vi "Trama_GGA(SubVI).vi"(0 "TRAMA":string) -> (1 "Cluster 2":T2, 2 "Cluster":T3, 3 "output":T1)   [LabVIEW 2020]
panel:
  out "String":string
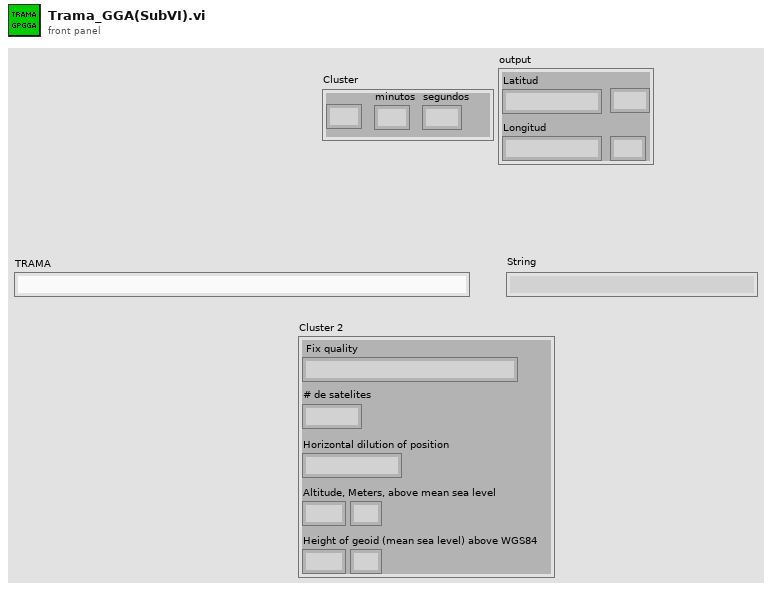
[diagram p1: front panel]
types:
  T1 = cluster{"Latitud":string, string, "Longitud":string, string}
  T2 = cluster{" Fix quality":string, "Horizontal dilution of position":string, "Altitude, Meters, above mean sea level":string, string, "Height of geoid (mean sea level) above WGS84":string, string, "# de satelites":string}
  T3 = cluster{"horas":string, "minutos":string, "segundos ":string}
  T4 = cluster{string, string, string, string, string, string, string}
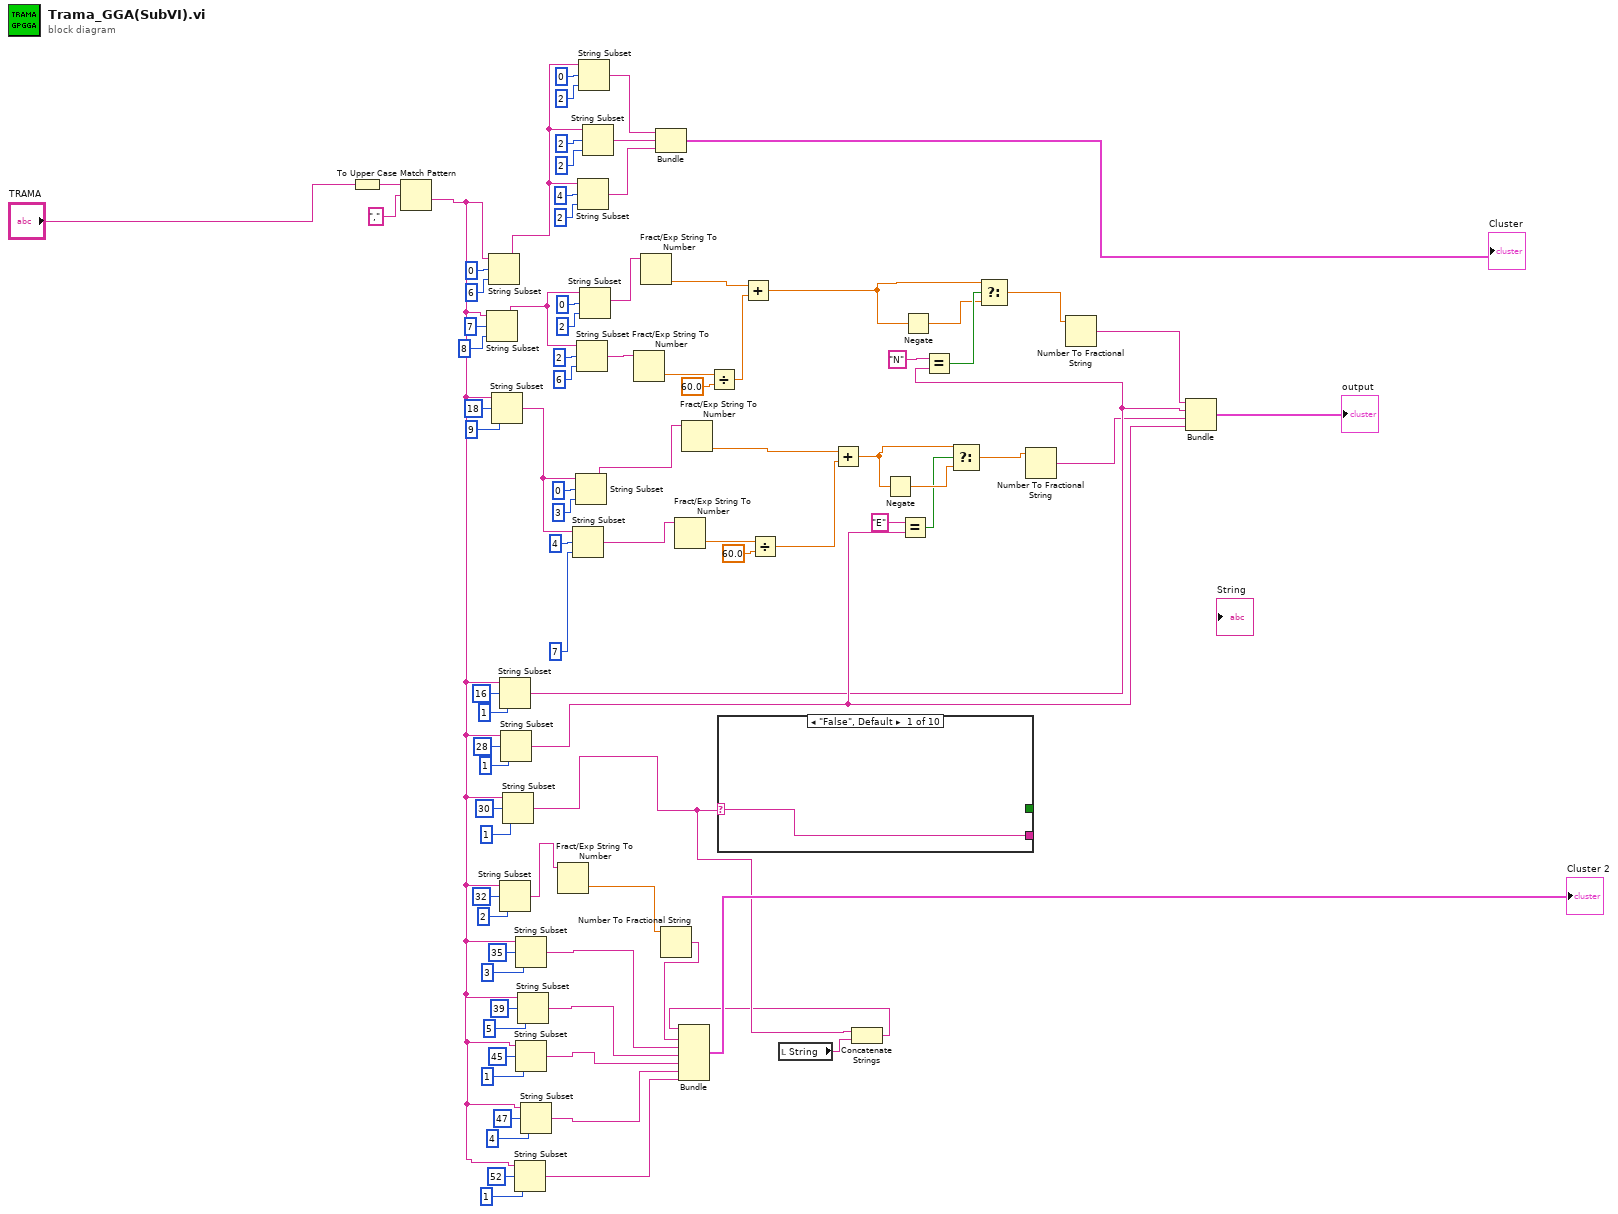
[diagram p0: block diagram]
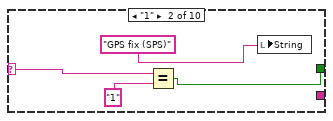
[diagram p2: hidden frame]
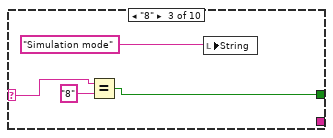
[diagram p3: hidden frame]
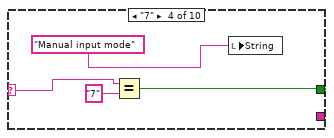
[diagram p4: hidden frame]
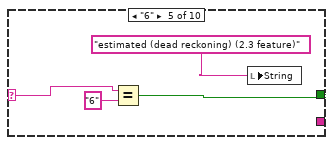
[diagram p5: hidden frame]
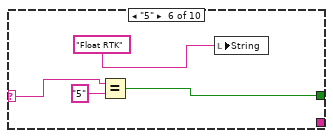
[diagram p6: hidden frame]
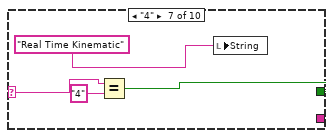
[diagram p7: hidden frame]
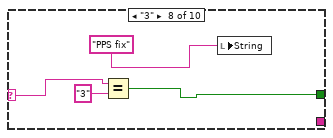
[diagram p8: hidden frame]
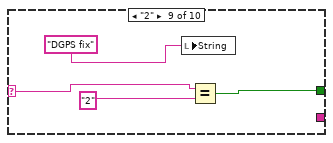
[diagram p9: hidden frame]
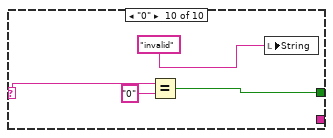
[diagram p10: hidden frame]
diagram:
  n1 = To Upper Case(1:"TRAMA") -> (0:w38:string)
  n2 = Match Pattern(string=w38, regular expression=",") -> (after substring=w80:string)  [unwired: 1 in, 3 out]
  n3 = String Subset(string=w80, offset (0)=7, length (rest)=8 ("length (rest)")) -> (substring=w35:string)
  n4 = String Subset(string=w80, offset (0)=0, length (rest)=6 ("length (rest)")) -> (substring=w37:string)
  n5 = String Subset(string=w80, offset (0)=18, length (rest)=9 ("length (rest)")) -> (substring=w51:string)
  n6 = String Subset(string=w80, offset (0)=16, length (rest)=1 ("length (rest)")) -> (substring=w58:string)
  n7 = String Subset(string=w80, offset (0)=32, length (rest)=2 ("length (rest)")) -> (substring=w87:string)
  n8 = String Subset(string=w80, offset (0)=28, length (rest)=1 ("length (rest)")) -> (substring=w65:string)
  n9 = String Subset(string=w80, offset (0)=30, length (rest)=1 ("length (rest)")) -> (substring=w10:string)
  n10 = String Subset(string=w80, offset (0)=52, length (rest)=1 ("length (rest)")) -> (substring=w85:string)
  n11 = String Subset(string=w80, offset (0)=35, length (rest)=3 ("length (rest)")) -> (substring=w81:string)
  n12 = String Subset(string=w80, offset (0)=45, length (rest)=1 ("length (rest)")) -> (substring=w83:string)
  n13 = String Subset(string=w80, offset (0)=39, length (rest)=5 ("length (rest)")) -> (substring=w82:string)
  n14 = String Subset(string=w80, offset (0)=47, length (rest)=4 ("length (rest)")) -> (substring=w84:string)
  n15 = Fract/Exp String To Number(string=w87) -> (number=w2:dbl)  [unwired: 3 in, 1 out]
  n16 = String Subset(string=w51, offset (0)=4, length (rest)=7 ("length (rest)")) -> (substring=w43:string)
  n17 = String Subset(string=w51, offset (0)=0, length (rest)=3 ("length (rest)")) -> (substring=w48:string)
  n18 = String Subset(string=w35, offset (0)=2, length (rest)=6 ("length (rest)")) -> (substring=w22:string)
  n19 = String Subset(string=w37, offset (0)=4, length (rest)=2 ("length (rest)")) -> (substring=w34:string)
  n20 = String Subset(string=w37, offset (0)=0, length (rest)=2 ("length (rest)")) -> (substring=w32:string)
  n21 = String Subset(string=w35, offset (0)=0, length (rest)=2 ("length (rest)")) -> (substring=w25:string)
  n22 = String Subset(string=w37, offset (0)=2, length (rest)=2 ("length (rest)")) -> (substring=w33:string)
  n23 = Fract/Exp String To Number(string=w22) -> (number=w23:dbl)  [unwired: 3 in, 1 out]
  n24 = Fract/Exp String To Number(string=w25) -> (number=w27:dbl)  [unwired: 3 in, 1 out]
  n25 = Bundle(w32, w33, w34) -> (→"Cluster":cluster{string, string, string})  [unwired: 1 in]
  n26 = Number To Fractional String(number=w2) -> (F-format string=w1:string)  [unwired: 3 in]
  n27 = Fract/Exp String To Number(string=w43) -> (number=w44:dbl)  [unwired: 3 in, 1 out]
  n28 = Fract/Exp String To Number(string=w48) -> (number=w47:dbl)  [unwired: 3 in, 1 out]
  n29 = Divide(x=w23, y=60.0) -> (x/y=w26:dbl)
  n30 = case shown="\"False\", Default" w10 {
    selector: w10 -> [w89 w91 w95 w98 w102 w106 w110 w115 w119 w124]
    tunnel: [w89 _ _ _ _ _ _ _ _ _] -> _
    tunnel: [_ w90 w94 w99 w103 w107 w111 w114 w118 w122] -> _
    frame "False", Default {
    }
    frame "1" {
      n31 = Equal?(x=w91, y="1") -> (x = y?=w90:bool)
      n32 = local write "String"("GPS fix (SPS)" ("Fix quiality 2")) -> ()
    }
    frame "8" {
      n33 = Equal?(x=w95, y="8") -> (x = y?=w94:bool)
      n34 = local write "String"("Simulation mode" ("Fix quiality 2")) -> ()
    }
    frame "7" {
      n35 = Equal?(x=w98, y="7") -> (x = y?=w99:bool)
      n36 = local write "String"("Manual input mode" ("Fix quiality 2")) -> ()
    }
    frame "6" {
      n37 = Equal?(x=w102, y="6") -> (x = y?=w103:bool)
      n38 = local write "String"("estimated (dead reckoning) (2.3 feature)" ("Fix quiality 2")) -> ()
    }
    frame "5" {
      n39 = Equal?(x=w106, y="5") -> (x = y?=w107:bool)
      n40 = local write "String"("Float RTK" ("Fix quiality 2")) -> ()
    }
    frame "4" {
      n41 = Equal?(x=w110, y="4") -> (x = y?=w111:bool)
      n42 = local write "String"("Real Time Kinematic" ("Fix quiality 2")) -> ()
    }
    frame "3" {
      n43 = Equal?(x=w115, y="3") -> (x = y?=w114:bool)
      n44 = local write "String"("PPS fix" ("Fix quiality 2")) -> ()
    }
    frame "2" {
      n45 = local write "String"("DGPS fix" ("Fix quiality 2")) -> ()
      n46 = Equal?(x=w119, y="2") -> (x = y?=w118:bool)
    }
    frame "0" {
      n47 = Equal?(x=w124, y="0") -> (x = y?=w122:bool)
      n48 = local write "String"("invalid" ("Fix quiality 2")) -> ()
    }
  }
  n49 = Add(x=w27, y=w26) -> (x+y=w56:dbl)
  n50 = Divide(x=w44, y=60.0) -> (x/y=w46:dbl)
  n51 = local read "String"() -> (w9:string)
  n52 = Add(x=w47, y=w46) -> (x+y=w64:dbl)
  n53 = Concatenate Strings(w10, w9) -> (w8:string)
  n54 = Bundle(w8, w1, w81, w82, w83, w84, w85) -> (→"Cluster 2":T4)  [unwired: 1 in]
  n55 = Negate(x=w64) -> (-x=w63:dbl)
  n56 = Equal?(x="E", y=w65) -> (x = y?=w61:bool)
  n57 = Negate(x=w56) -> (-x=w57:dbl)
  n58 = Equal?(x="N", y=w58) -> (x = y?=w60:bool)
  n59 = Select(t=w64, s=w61, f=w63) -> (s? t:f=w7:dbl)
  n60 = Select(t=w56, s=w60, f=w57) -> (s? t:f=w4:dbl)
  n61 = Number To Fractional String(number=w7) -> (F-format string=w6:string)  [unwired: 3 in]
  n62 = Number To Fractional String(number=w4) -> (F-format string=w5:string)  [unwired: 3 in]
  n63 = Bundle(w5, w58, w6, w65) -> (→"output":cluster{string, string, string, string})  [unwired: 1 in]
